vi "Control Valve Smoothing.vi"(10 "CV Control Voltages":dbl[](array[numeric]), 11 "Averaged In":dbl[][](array[numeric])) -> (2 "Smoothed Voltage":dbl[](array[numeric]), 3 "Averaged Out":dbl[][](array[numeric]))   [LabVIEW 2018]
uses:
  <vilib>/Analysis/baseanly.llb/Mean (DBL).vi
  <vilib>/Analysis/NI_AALBase.lvlib
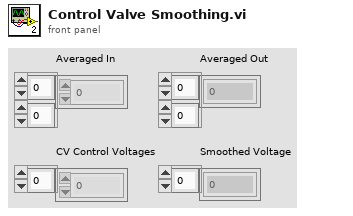
[diagram p1: front panel]
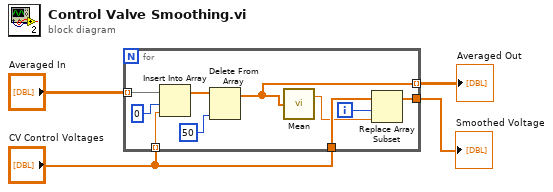
[diagram p0: block diagram]
diagram:
  n1 = for {
    tunnel: "Averaged In" -> [w14] mode=indexing
    tunnel: "CV Control Voltages" -> [w13] mode=indexing
    tunnel: "CV Control Voltages" -> [w9]
    tunnel: [w6] -> w3
    tunnel: [w5] -> w4 mode=indexing
    i -> [w7]
    n2 = Insert Into Array(array=w14, index=0, new element=w13) -> (w11:dbl[])
    n3 = Delete From Array(array=w11, index=50) -> (array with subset deleted=w5:dbl[])  [unwired: 1 in, 1 out]
    n4 = call-poly <vilib>:"Mean.vi"("X"=w5) -> ("mean"=w8:dbl)  [unwired: 1 out]
    n5 = Replace Array Subset(array=w9, new element=w8, index=w7) -> (w6:dbl[])
  }
  "Averaged Out" <- w4
  "Smoothed Voltage" <- w3
